vi "DisableControls.vi"(0 "Operation Interface in":refnum<class "Operation Interface.lvclass">, 5 "error in (no error)":errorcluster) -> (14 "Operation Interface out":refnum<class "Operation Interface.lvclass">, 19 "error out":errorcluster)   [LabVIEW 2016, in "Operation Interface.lvclass"]
uses:
  Operation Interface.lvclass
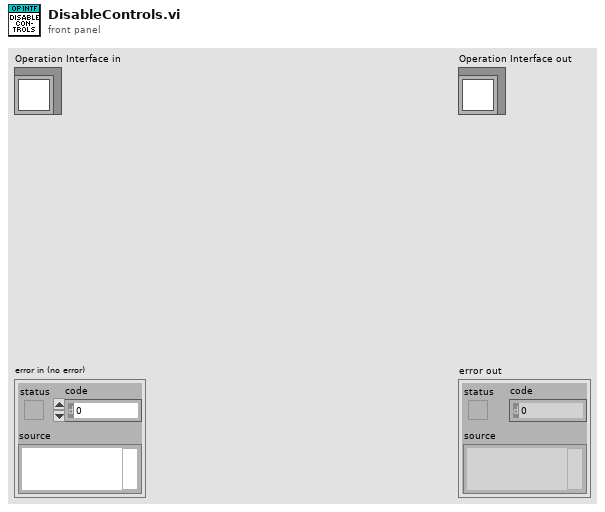
[diagram p1: front panel]
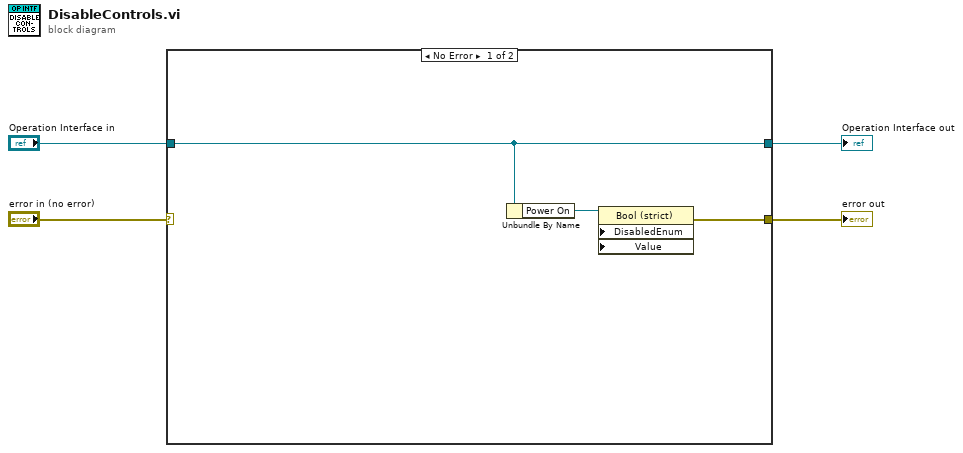
[diagram p0: block diagram]
diagram:
  n1 = case shown="No Error" "error in (no error)" {
    selector: "error in (no error)" -> [_ w9]
    tunnel: [w5 w9] -> w3
    tunnel: [w7 w8] -> w1
    tunnel: "Operation Interface in" -> [w7 w8]
    frame No Error {
      n2 = Unbundle By Name(w7) -> ("Power On"=w6:refnum<vi>)
      n3 = property class="Bool (strict)" props=["DisabledEnum", "Value"](reference=w6) -> (error out=w5:errorcluster)  [unwired: 3 in, 1 out]
    }
    frame Error {
    }
  }
  "error out" <- w3
  "Operation Interface out" <- w1
